vi "Encapsulate.vi"(8 "error in (no error)":errorcluster, 9 "size":u64 format="%d bytes", 10 "address":u64 format="%016x", 11 "Pointer type":refnum<class "Pointer.lvclass">) -> (0 "error out":errorcluster, 3 "Pointer out":refnum<class "Pointer.lvclass">)   [LabVIEW 2016, in "Memory Manager.lvlib" / "Pointer.lvclass"]
doc: "Encapsulates an existing pointer allocated externally to LabVIEW to allow manipulation of that pointer using this library."
uses:
  Pointer.lvclass
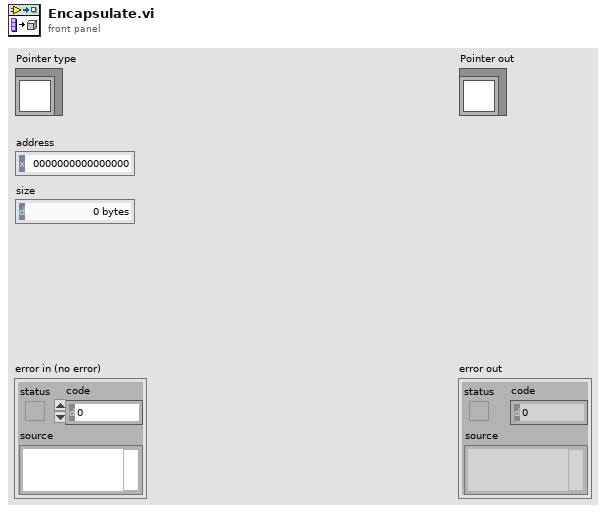
[diagram p1: front panel]
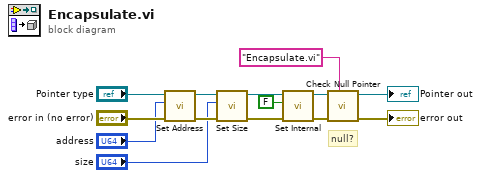
[diagram p0: block diagram]
diagram:
  # "null?"
  n1 = call "Set Address.vi"("address"="address", "Pointer in"="Pointer type") -> ("Pointer out"=w10:refnum<class "Pointer.lvclass">)  [unwired: 9 in]
  n2 = call "Set Size.vi"("size"="size", "Pointer in"=w10) -> ("Pointer out"=w1:refnum<class "Pointer.lvclass">)  [unwired: 9 in]
  n3 = call "Set Internal.vi"("internal"=FALSE, "Pointer in"=w1) -> ("Pointer out"=w2:refnum<class "Pointer.lvclass">)  [unwired: 9 in]
  n4 = call "Check Null Pointer.vi"("source vi name"="Encapsulate.vi", "error in (no error)"="error in (no error)", "Pointer in"=w2) -> ("error out"=→"error out":errorcluster, "Pointer out"=→"Pointer out":refnum<class "Pointer.lvclass">)  [unwired: 7 in]
